vi "Control Digital Output - PWM - Update Frequency.vi"(0 "frequency":dbl=1.0 format="%.6f", 5 "duty cycle":dbl=0.5 format="%.6f", 7 "task in":refnum<k21>, 11 "Error In":errorcluster) -> (4 "task out":refnum<k21>, 15 "Error Out":errorcluster)   [LabVIEW 2016]
uses:
  <resource>/objmgr/daqmx.rc
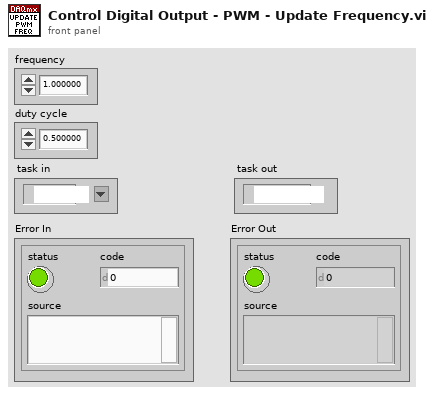
[diagram p1: front panel]
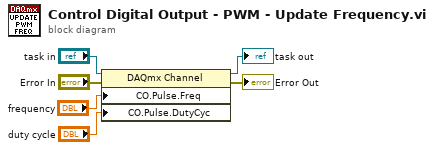
[diagram p0: block diagram]
diagram:
  n1 = property class="DAQmx Channel"(reference="task in", error in="Error In", "CO.Pulse.Freq"="frequency", "CO.Pulse.DutyCyc"="duty cycle") -> (reference out=→"task out":refnum<k21>, error out=→"Error Out":errorcluster)
